vi "Dequeue.vi"(6 "timeout in ms (-1)":i32=-1, 8 "error in (no error)":errorcluster, 11 "Message Queue":refnum<queue>) -> (0 "error out":errorcluster, 1 "Message Data":variant, 2 "State":T1, 3 "dup Message Queue":refnum<queue>, 4 "timed out?":bool, 5 "Call Chain":string[](array[string]))   [LabVIEW 2019, in "Status.lvlib"]
doc: "This VI pulls messages off the Message Queue."
uses:
  Status.lvlib
  Queue Type.ctl
  State Name.ctl
  4c130db5-5630-4b43-ac4a-385984f4c958.vi
panel:
  out "# elements in queue":i32
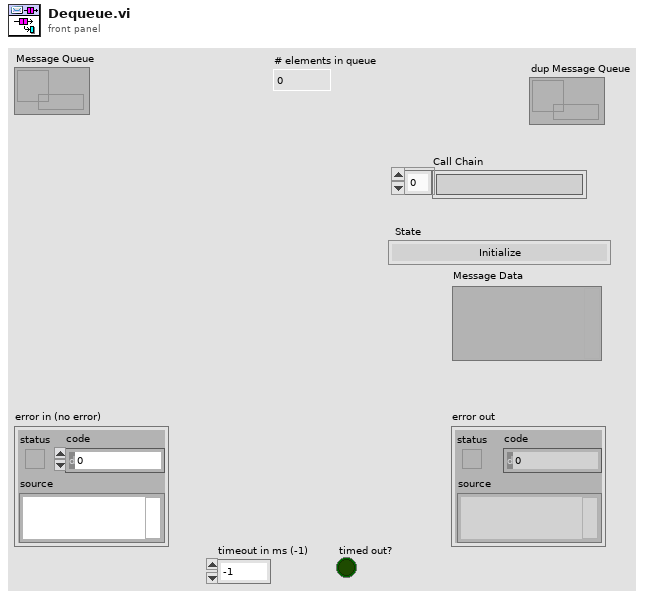
[diagram p1: front panel]
types:
  T1 = typedef "Status.lvlib/State Name.ctl" = enum16{"Initialize", "Update Progress Bar", "Update Status Bar", "Set Cursor Busy", "Unset Cursor Busy", "Error", "Default", "Exit"}
  T2 = typedef "Status.lvlib/Queue Type.ctl" = cluster{"Custom State Name":string, "Defined State Name":T1, "Call Chain":string[], "Message Data":variant}
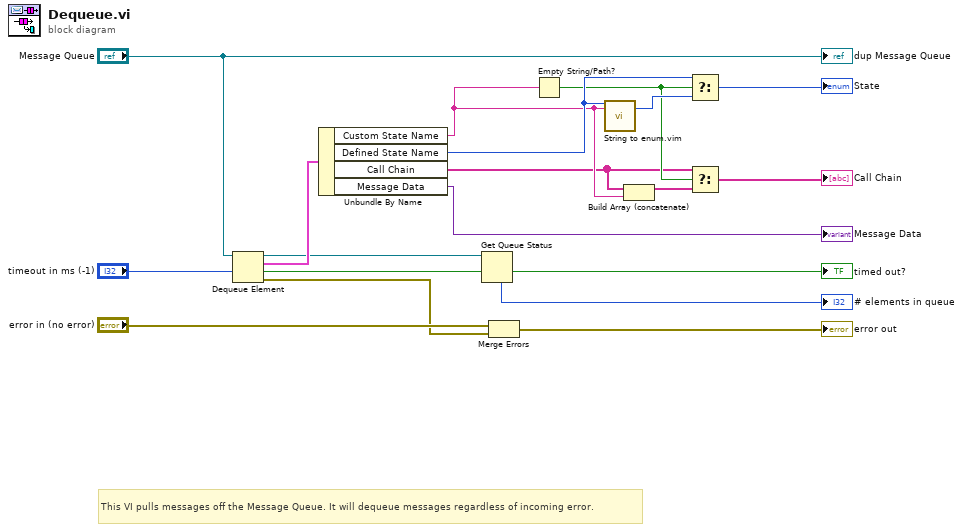
[diagram p0: block diagram]
diagram:
  # "This VI pulls messages off the Message Queue. It will dequeue messages regardless of incoming error."
  n1 = Dequeue Element(queue="Message Queue", timeout in ms (-1)="timeout in ms (-1)") -> (queue out=w13:refnum<queue>, element=w18:T2, timed out?=→"timed out?":bool, error out=w15:errorcluster)  [unwired: 1 in]
  n2 = Unbundle By Name(w18) -> ("Custom State Name"=w5:string, "Defined State Name"=w8:T1, "Call Chain"=w3:string[], "Message Data"=→"Message Data":variant)
  n3 = Get Queue Status(queue=w13) -> (# elements in queue=→"# elements in queue":i32)  [unwired: 2 in, 7 out]
  n4 = Merge Errors("error in (no error)", w15) -> (→"error out":errorcluster)
  n5 = Empty String/Path?(string/path=w5) -> (empty?=w4:bool)
  n6 = call "String to enum.vim"("Enum"=w8, "Item Name"=w5) -> ("Enum Selected"=w7:u16)  [unwired: 15 in, 2 out]
  n7 = Build Array (concatenate)(w3, w5) -> (w2:string[])
  n8 = Select(t=w8, s=w4, f=w7) -> (s? t:f=→"State":u16)
  n9 = Select(t=w3, s=w4, f=w2) -> (s? t:f=→"Call Chain":string[])
  "dup Message Queue" <- "Message Queue"
